vi "ESCON_505_Controller.vi"(1 "u":dbl) -> (0 "Modified u":i16)   [LabVIEW 2019]
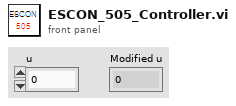
[diagram p1: front panel]
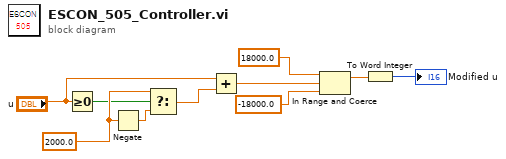
[diagram p0: block diagram]
diagram:
  w7 = 2000.0
  n1 = Greater Or Equal To 0?(x="u") -> (x >= 0?=w6:bool)
  n2 = Negate(x=w7) -> (-x=w8:dbl)
  n3 = Select(t=w7, s=w6, f=w8) -> (s? t:f=w9:dbl)
  n4 = Add(x="u", y=w9) -> (x+y=w5:dbl)
  n5 = In Range and Coerce(upper limit=18000.0, x=w5, lower limit=-18000.0) -> (coerced(x)=w2:dbl)  [unwired: 1 out]
  n6 = To Word Integer(number=w2) -> (16bit integer=→"Modified u":i16)
